vi "FGV.Main.vi"() -> ()   [LabVIEW 2009, in "HB_BaseClass_Examples.lvlib"]
doc: "This VI demonstrates the usage of HGF_FGV."
uses:
  HB_BaseClass_Examples.lvlib
  lib.lib/HGF_LVC/HGF_BaseClasses/HGF_FGV/HGF_FGV_Append/HGF_FGV_Append.lvclass
  HB_Simple/Visitors/Increment/HB_Simple_Increment.lvclass
  lib.lib/HGF_LVC/HGF_BaseClasses/HGF_FGV/HGF_FGV_VisitAll/HGF_FGV_VisitAll.lvclass
  lib.lib/HGF_LVC/HGF_BaseClasses/HGF_FGV/HGF_FGV_Subset/HGF_FGV_SubSet.lvclass
  HB_Simple/HB_Simple.lvclass
  lib.lib/HGF_LVC/HGF_BaseClasses/HGF_FGV/HGF_FGV_Clear/HGF_FGV_Clear.lvclass
  lib.lib/HGF_LVC/HGF_BaseClasses/HGF_FGV/HGF_FGV_Factory/HGF_FGV_Factory.lvclass
  HB_Factory/HB_Factory.lvclass
  lib.lib/HGF_LVC/HGF_BaseClasses/HGF_Factory/HGF_Factory.lvclass
  lib.lib/HGF_LVC/HGF_BaseClasses/HGF_FGV/HGF_FGV_Visitor/HGF_FGV_Visitor.lvclass
panel:
  out "nofObjects":i32
  out "x Array":dbl[](array[numeric])
  out "initData Found?":bool
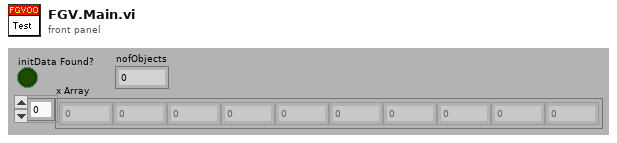
[diagram p1: front panel]
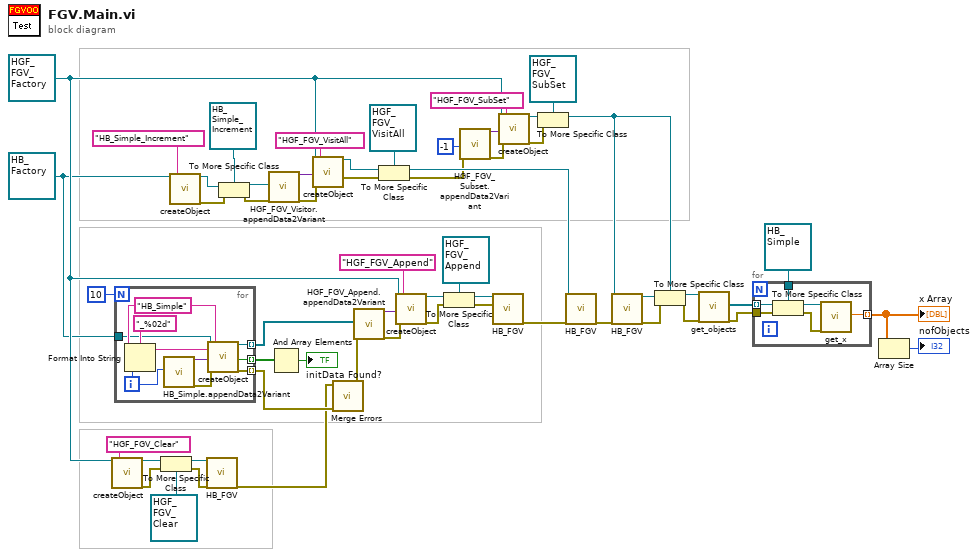
[diagram p0: block diagram]
diagram:
  w1 = refnum<class "HB_Factory.lvclass"> refnum ("HB_HGF_Test.lvlib:HB_Factory.lvclass")
  w2 = refnum<class "HGF_FGV_Factory.lvclass"> refnum ("HGF_FGV.lvlib:HGF_FGV_Factory.lvclass")
  n1 = call "createObject.vi"("HGF_Factory"=w2, "className"="HGF_FGV_Clear") -> ("HGF_Object"=w3:refnum<class "HGF_Factory.lvclass">, "error out"=w15:errorcluster)  [unwired: 3 in, 13 out]
  n2 = for {
    N: 10 -> [_]
    tunnel: w1 -> [w61]
    tunnel: [w60] -> w56 mode=indexing
    tunnel: [w59] -> w55 mode=indexing
    tunnel: [w57] -> w50 mode=indexing
    i -> [w58]
    w64 = "HB_Simple" ("className")
    n3 = Format Into String(format string="_%02d", initial string=w64, w58) -> (resulting string=w63:string)  [unwired: 1 in, 1 out]
    n4 = call "HB_Simple.appendData2Variant.vi"("x"=w58) -> ("dup initData"=w66:variant, "error out"=w65:errorcluster)  [unwired: 17 in]
    n5 = call "createObject.vi"("HGF_Factory"=w61, "objectName"=w63, "initializationData"=w66, "error in (no error)"=w65, "className"=w64) -> ("HGF_Object"=w57:refnum<class "HGF_Factory.lvclass">, "found?"=w60:bool, "error out"=w59:errorcluster)  [unwired: 12 out]
  }
  n6 = To More Specific Class(target class=refnum<class "HGF_FGV_Clear.lvclass"> refnum ("HGF_FGV.lvlib:HGF_FGV_Clear.lvclass"), reference=w3, error in=w15) -> (specific class reference=w13:refnum<class "HGF_FGV_Clear.lvclass">, error out=w12:errorcluster)
  n7 = call "createObject.vi"("HGF_Factory"=w1, "className"="HB_Simple_Increment") -> ("HGF_Object"=w7:refnum<class "HGF_Factory.lvclass">, "error out"=w44:errorcluster)  [unwired: 3 in, 13 out]
  n8 = call "HB_FGV.vi"("HGF_FGV_Action"=w13, "error in (no error)"=w12) -> ("error out"=w8:errorcluster)  [unwired: 17 out]
  n9 = To More Specific Class(target class=refnum<class "HB_Simple_Increment.lvclass"> refnum ("HGF_BaseClass_Examples.lvlib:HB_Simple_Increment.lvclass"), reference=w7, error in=w44) -> (specific class reference=w42:refnum<class "HB_Simple_Increment.lvclass">, error out=w41:errorcluster)
  n10 = call "HGF_FGV_Visitor.appendData2Variant.vi"("HGF_Visitor"=w42, "error in (no error)"=w41) -> ("dup initData"=w40:variant, "error out"=w38:errorcluster)  [unwired: 1 in, 15 out]
  n11 = And Array Elements(Boolean array=w56) -> (logical AND=→"initData Found?":bool)
  n12 = call "createObject.vi"("HGF_Factory"=w2, "initializationData"=w40, "error in (no error)"=w38, "className"="HGF_FGV_VisitAll") -> ("HGF_Object"=w5:refnum<class "HGF_Factory.lvclass">, "error out"=w37:errorcluster)  [unwired: 2 in, 12 out]
  n13 = call <vilib>:"Merge Errors.vi"("error array in"=w55, "error in 1 (no error)"=w8) -> ("error out"=w48:errorcluster)  [unwired: 2 in, 3 out]
  n14 = call "HGF_FGV_Append.appendData2Variant.vi"("Objects"=w50, "error in (no error)"=w48) -> ("dup initData"=w52:variant, "error out"=w51:errorcluster)  [unwired: 1 in, 15 out]
  n15 = To More Specific Class(target class=refnum<class "HGF_FGV_VisitAll.lvclass"> refnum ("HGF_FGV.lvlib:HGF_FGV_VisitAll.lvclass"), reference=w5, error in=w37) -> (specific class reference=w35:refnum<class "HGF_FGV_VisitAll.lvclass">, error out=w30:errorcluster)
  n16 = call "createObject.vi"("HGF_Factory"=w2, "initializationData"=w52, "error in (no error)"=w51, "className"="HGF_FGV_Append") -> ("HGF_Object"=w4:refnum<class "HGF_Factory.lvclass">, "error out"=w46:errorcluster)  [unwired: 1 in, 13 out]
  n17 = To More Specific Class(target class=refnum<class "HGF_FGV_Append.lvclass"> refnum ("HGF_FGV.lvlib:HGF_FGV_Append.lvclass"), reference=w4, error in=w46) -> (specific class reference=w45:refnum<class "HGF_FGV_Append.lvclass">, error out=w9:errorcluster)
  n18 = call "HGF_FGV_Subset.appendData2Variant.vi"("length"=-1, "error in (no error)"=w30) -> ("dup initData"=w32:variant, "error out"=w29:errorcluster)  [unwired: 2 in, 14 out]
  n19 = call "HB_FGV.vi"("HGF_FGV_Action"=w45, "error in (no error)"=w9) -> ("error out"=w11:errorcluster)  [unwired: 17 out]
  n20 = call "createObject.vi"("HGF_Factory"=w2, "initializationData"=w32, "error in (no error)"=w29, "className"="HGF_FGV_SubSet") -> ("HGF_Object"=w6:refnum<class "HGF_Factory.lvclass">, "error out"=w28:errorcluster)  [unwired: 1 in, 13 out]
  n21 = To More Specific Class(target class=refnum<class "HGF_FGV_SubSet.lvclass"> refnum ("HGF_FGV.lvlib:HGF_FGV_SubSet.lvclass"), reference=w6, error in=w28) -> (specific class reference=w24:refnum<class "HGF_FGV_SubSet.lvclass">)  [unwired: 1 out]
  n22 = call "HB_FGV.vi"("HGF_FGV_Action"=w35, "error in (no error)"=w11) -> ("error out"=w10:errorcluster)  [unwired: 17 out]
  n23 = call "HB_FGV.vi"("HGF_FGV_Action"=w24, "error in (no error)"=w10) -> ("dup HGF_FGV_Action"=w26:refnum<class "HGF_FGV_SubSet.lvclass">, "error out"=w25:errorcluster)  [unwired: 16 out]
  n24 = To More Specific Class(target class=w24, reference=w26, error in=w25) -> (specific class reference=w23:refnum<class "HGF_FGV_SubSet.lvclass">, error out=w22:errorcluster)
  n25 = call "get_objects.vi"("HGF_FGV_Subset"=w23, "error in (no error)"=w22) -> ("Objects"=w21:refnum<class>[], "error out"=w20:errorcluster)  [unwired: 16 out]
  n26 = for {
    tunnel: w21 -> [w71] mode=indexing
    tunnel: w20 -> [w70]
    tunnel: refnum<class "HB_Simple.lvclass"> refnum ("HGF_BaseClass_Examples.lvlib:HB_Simple.lvclass") -> [w68]
    tunnel: [w67] -> w18 mode=indexing
    n27 = To More Specific Class(target class=w68, reference=w71, error in=w70) -> (specific class reference=w72:refnum<class "HB_Simple.lvclass">, error out=w69:errorcluster)
    n28 = call "get_x.vi"("HB_Simple"=w72, "error in (no error)"=w69) -> ("x"=w67:dbl)  [unwired: 17 out]
  }
  "x Array" <- w18
  n29 = Array Size(array=w18) -> (size(s)=→"nofObjects":i32)
